vi "Pockels-Convert AO sequence from samples to time.vi"(11 "Number of samples in AO sequence":i32) -> (3 "Duration of AO sequence (us)":dbl format="%#_6f")   [LabVIEW 2020]
uses:
  Global Variables/General Globals.vi
panel:
  out "Sampling period (us)":dbl
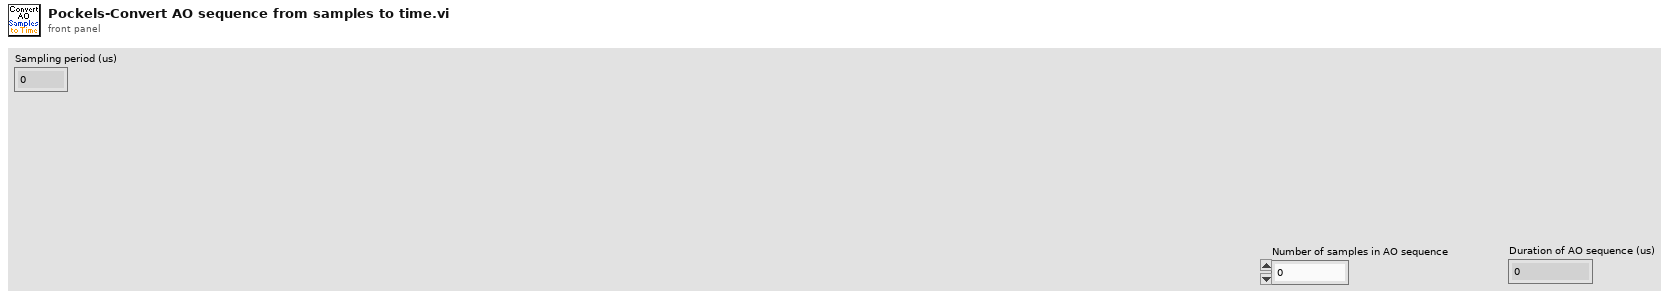
[diagram p1: front panel]
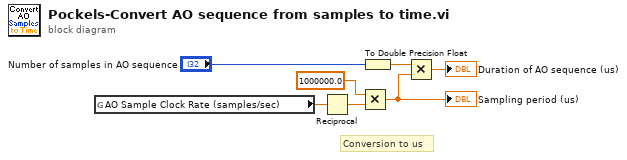
[diagram p0: block diagram]
diagram:
  # "Conversion to us"
  n1 = global read "General Globals.vi" "AO Sample Clock Rate (samples/sec)"() -> (w5:dbl)
  n2 = Reciprocal(x=w5) -> (1/x=w7:dbl)
  n3 = Multiply(x=1000000.0 ("y"), y=w7) -> (x*y=w4:dbl)
  "Sampling period (us)" <- w4
  n4 = To Double Precision Float(number="Number of samples in AO sequence") -> (double precision float=w1:dbl)
  n5 = Multiply(x=w1, y=w4) -> (x*y=→"Duration of AO sequence (us)":dbl)
